vi "LEDControl.vi"() -> ()   [LabVIEW 2022 SP3]
panel:
  in  "POWER SUPPLY":refnum<visa-resource-name>
  out "CURRENT VALUE\n (mA)":dbl
  in  "STOP BUTTON":bool
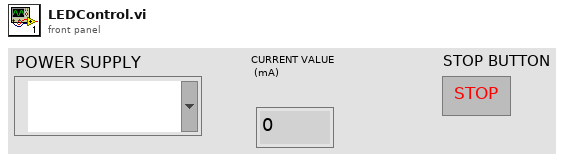
[diagram p1: front panel]
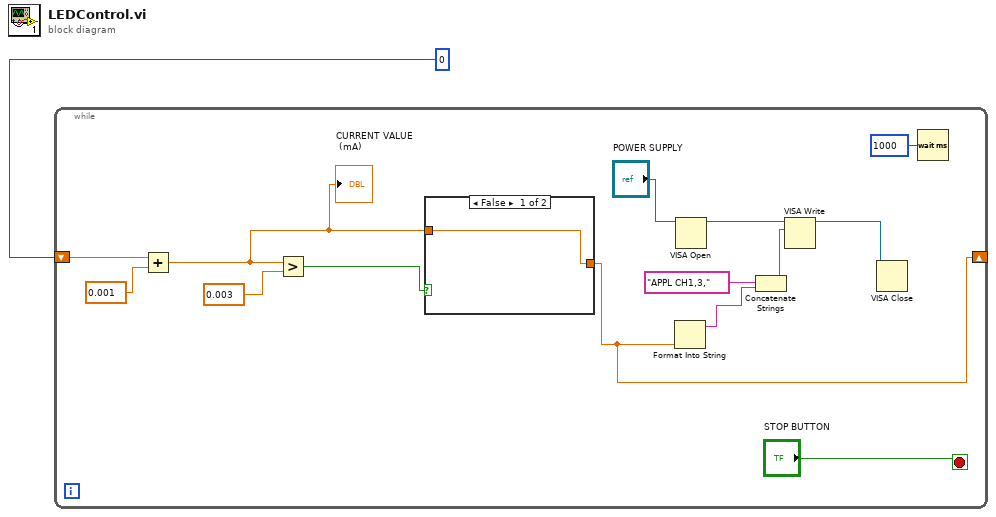
[diagram p0: block diagram]
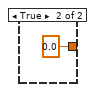
[diagram p2: hidden frame]
diagram:
  n1 = while {
    shift-right: [w2] -> _
    shift-left: 0 -> [w13]
    stop <- "STOP BUTTON" stop-if-true
    n2 = Add(x=w13, y=0.001) -> (x+y=w11:dbl)
    "CURRENT VALUE\n (mA)" <- w11
    n3 = Greater?(x=w11, y=0.003) -> (0:w12:bool)
    n4 = case shown="False" w12 {
      tunnel: [w16 0.0] -> w2
      tunnel: w11 -> [w16 _]
      frame False {
      }
      frame True {
      }
    }
    n5 = Format Into String(w2) -> (resulting string=w6:string)  [unwired: 3 in, 1 out]
    n6 = VISA Open(VISA resource name="POWER SUPPLY") -> (VISA resource name=w10:refnum<visa-resource-name>)  [unwired: 4 in, 1 out]
    n7 = Concatenate Strings("APPL CH1,3," ("write buffer"), w6) -> (w5:string)
    n8 = VISA Write(VISA resource name=w10, write buffer=w5) -> (VISA resource name out=w9:refnum<visa-resource-name>)  [unwired: 1 in, 2 out]
    n9 = VISA Close(VISA resource name=w9) -> ()  [unwired: 1 in, 1 out]
    n10 = Wait (ms)(milliseconds to wait=u32 1000) -> ()  [unwired: 1 out]
  }
